vi "S2C_FORNAX_Proc_FindFnxMsgs.vi"(8 "Error In":errorcluster, 11 "MsgName":string) -> (0 "Error Out":errorcluster, 3 "Messages":string[](array[string]))   [LabVIEW 2015]
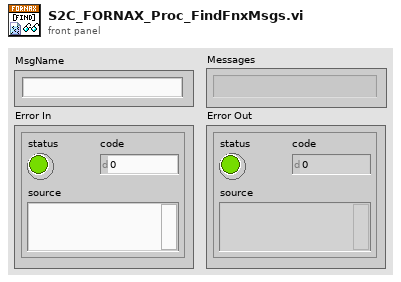
[diagram p1: front panel]
types:
  T1 = cluster{"RawMsg":string, "ViperMsg":string[], "DDSMsg":string[]}
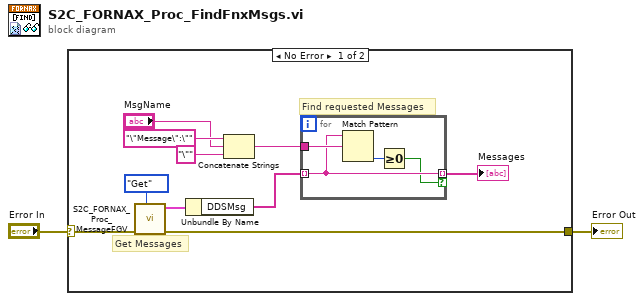
[diagram p0: block diagram]
diagram:
  n1 = case shown="No Error" "Error In" {
    selector: "Error In" -> [w12 w17]
    tunnel: [w4 w17] -> w1
    frame No Error {
      # "Find requested Messages"
      # "Get Messages"
      n2 = call "S2C_FORNAX_Proc_MessageFGV.vi"("Action"=enum16{"Set", "Get"}."Get", "Error In"=w12) -> ("Error Out"=w4:errorcluster, "Msg Out"=w7:T1)  [unwired: 8 in]
      n3 = Unbundle By Name(w7) -> ("DDSMsg"=w6:string[])
      n4 = Concatenate Strings("\"Message\":\"" ("regular expression"), "MsgName", "\"" ("regular expression")) -> (w5:string)
      n5 = for {
        tunnel: w6 -> [w14] mode=indexing
        tunnel: w5 -> [w16]
        tunnel: [w14] -> w3 mode=indexing if=w13
        n6 = Match Pattern(string=w14, regular expression=w16) -> (offset past match=w15:i32)  [unwired: 1 in, 3 out]
        n7 = Greater Or Equal To 0?(x=w15) -> (x >= 0?=w13:bool)
      }
      "Messages" <- w3
    }
    frame Error {
    }
  }
  "Error Out" <- w1
